vi "L13.vi"() -> ()   [LabVIEW 2012]
panel:
  out "add":string
  out "add 10":string
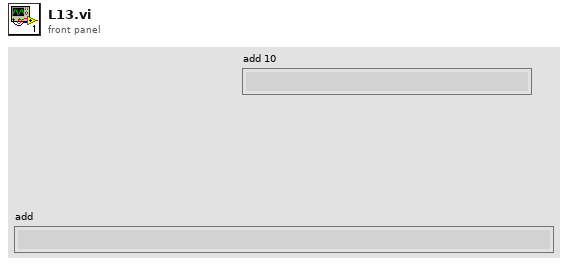
[diagram p1: front panel]
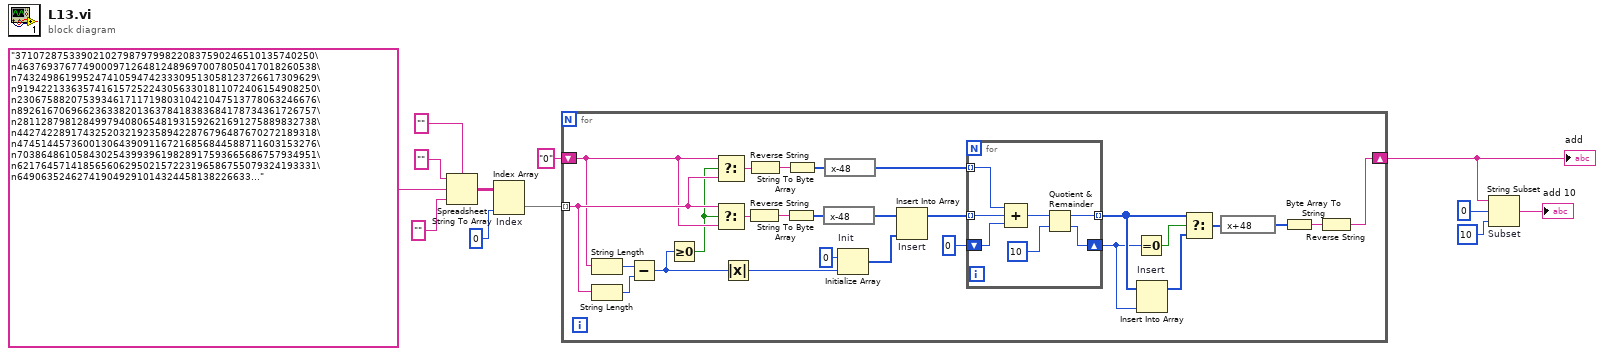
[diagram p0: block diagram]
diagram:
  n1 = Spreadsheet String To Array(delimiter (Tab)="", format string="", spreadsheet string="37107287533902102798797998220837590246510135740250\n46376937677490009712648124896970078050417018260538\n74324986199524741059474233309513058123726617309629\n91942213363574161572522430563301811072406154908250\n23067588207539346171171980310421047513778063246676\n89261670696623633820136378418383684178734361726757\n28112879812849979408065481931592621691275889832738\n44274228917432520321923589422876796487670272189318\n47451445736001306439091167216856844588711603153276\n70386486105843025439939619828917593665686757934951\n62176457141856560629502157223196586755079324193331\n649063524627419049291014324458138226633...", array type (2D Dbl)="") -> (array=w8:string[][])
  n2 = Index Array "Index"(array=w8, index (col)=0 ("disabled index (col)")) -> (element=w6:string[])  [unwired: 1 in]
  n3 = for {
    tunnel: w6 -> [w19] mode=indexing
    shift-right: [w20] -> w4
    shift-left: "0" -> [w18]
    n4 = String Length(string=w18) -> (length=w34:i32)
    n5 = String Length(string=w19) -> (length=w33:i32)
    n6 = Subtract(x=w34, y=w33) -> (x-y=w14:i32)
    n7 = Greater Or Equal To 0?(x=w14) -> (x >= 0?=w17:bool)
    n8 = Select(t=w18, s=w17, f=w19) -> (s? t:f=w16:string)
    n9 = Select(t=w19, s=w17, f=w18) -> (s? t:f=w15:string)
    n10 = Absolute Value(x=w14) -> (abs(x)=w13:i32)
    n11 = Reverse String(1:w15) -> (0:w22:string)
    n12 = Reverse String(1:w16) -> (0:w21:string)
    n13 = String To Byte Array(string=w22) -> (unsigned byte array=w24:u8[])
    n14 = String To Byte Array(string=w21) -> (unsigned byte array=w23:u8[])
    n15 = expression code="x-48"(w24) -> (w31:u8[])
    n16 = expression code="x-48"(w23) -> (w32:u8[])
    n17 = Initialize Array "Init"(0 ("element"), w13) -> (w26:i32[])
    n18 = Insert Into Array "Insert"(array=w31, new element=w26) -> (w27:u8[])  [unwired: 1 in]
    n19 = for {
      tunnel: w27 -> [w42] mode=indexing
      tunnel: [w46] -> w38 mode=indexing
      shift-right: [w44] -> w37
      shift-left: u8 0 -> [w41]
      tunnel: w32 -> [w43] mode=indexing
      n20 = Compound Arithmetic op=ADD(w43, w42, w41) -> (w40:u8)
      n21 = Quotient & Remainder(x=w40, y=u8 10) -> (x-y*floor(x/y)=w46:u8, floor(x/y)=w44:u8)
    }
    n22 = Equal To 0?(x=w37) -> (x = 0?=w36:bool)
    n23 = Insert Into Array "Insert"(array=w38, new element=w37) -> (w35:u8[])  [unwired: 1 in]
    n24 = Select(t=w38, s=w36, f=w35) -> (s? t:f=w39:u8[])
    n25 = expression code="x+48"(w39) -> (w29:u8[])
    n26 = Byte Array To String(unsigned byte array=w29) -> (string=w30:string)
    n27 = Reverse String(1:w30) -> (0:w20:string)
  }
  "add" <- w4
  n28 = String Subset "Subset"(string=w4, offset (0)=0, length (rest)=10 ("length (rest)")) -> (substring=→"add 10":string)
